vi "写入数据.vi"(6 "数据属性":variant, 8 "错误输入（无错误）":errorcluster, 11 "测试数据":dbl[][](array[numeric])) -> (0 "错误输出":errorcluster)   [LabVIEW 2020]
uses:
  <vilib>/drjdpowell/SQLite Library/SQL Statement/SQL Statement.lvclass/SQL Statement.ctl
  <vilib>/drjdpowell/SQLite Library/SQL Connection/Open (path).vi
  <vilib>/drjdpowell/SQLite Library/SQL Statement/First Step.vi
  <vilib>/drjdpowell/SQLite Library/SQL Statement/Bind Timestamp (Real).vi
  <vilib>/drjdpowell/SQLite Library/SQL Statement/Bind Text.vi
  <vilib>/drjdpowell/SQLite Library/SQL Statement/Bind Blob.vi
  <vilib>/drjdpowell/SQLite Library/SQL Statement/Bind Integer.vi
  <vilib>/drjdpowell/SQLite Library/SQL Statement/Finalize (Property).vi
  <vilib>/drjdpowell/SQLite Library/SQL Connection/Open (string).vi
  <vilib>/drjdpowell/SQLite Library/SQL Statement/Step.vi
  <vilib>/drjdpowell/SQLite Library/SQL Statement/Bind Real.vi
  <vilib>/drjdpowell/SQLite Library/SQL Statement/Finalize.vi
  <vilib>/AdvancedString/Path To Command Line String.vi
  <vilib>/drjdpowell/SQLite Library/SQL Statement/Error Message.vi
  <vilib>/drjdpowell/SQLite Library/SQL Connection/Connection.lvclass
  <vilib>/drjdpowell/SQLite Library/SQL Statement/SQL Statement.lvclass
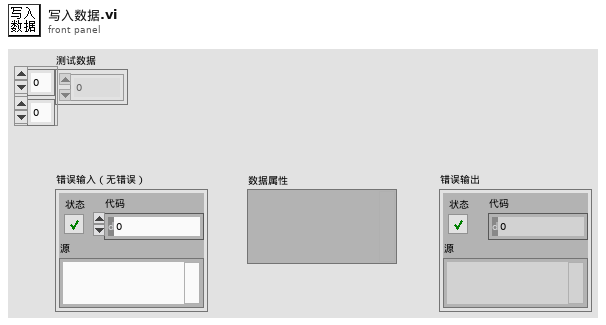
[diagram p1: front panel]
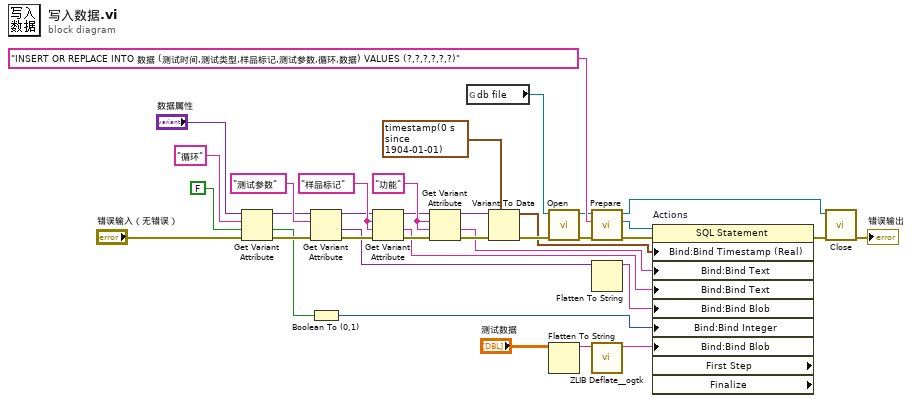
[diagram p0: block diagram]
diagram:
  w26 = "功能" ("元素")
  w33 = "样品标记" ("名称")
  n1 = Get Variant Attribute(Variant="数据属性", name="循环" ("名称"), default value (empty Variant)=FALSE, error in="错误输入（无错误）") -> (duplicate Variant=w24:variant, value=w6:bool, error out=w23:errorcluster)  [unwired: 1 out]
  n2 = Get Variant Attribute(Variant=w24, name="测试参数" ("元素"), error in=w23) -> (duplicate Variant=w22:variant, value=w8:variant, error out=w21:errorcluster)  [unwired: 1 in, 1 out]
  n3 = Boolean To (0,1)(Boolean=w6) -> (0, 1=w5:i16)
  n4 = Get Variant Attribute(Variant=w22, name=w33, default value (empty Variant)=w33, error in=w21) -> (duplicate Variant=w20:variant, value=w9:string, error out=w19:errorcluster)  [unwired: 1 out]
  n5 = Get Variant Attribute(Variant=w20, name=w26, default value (empty Variant)=w26, error in=w19) -> (duplicate Variant=w17:variant, value=w10:string, error out=w16:errorcluster)  [unwired: 1 out]
  n6 = global read "数据库.vi" "db file"() -> (w36:path)
  n7 = Variant To Data(error in=w16, type=timestamp(0 s since 1904-01-01), Variant=w17) -> (data=w11:timestamp, error out=w13:errorcluster)
  n8 = call-poly <vilib>:"Open.vi"("error in (no error)"=w13, "db file"=w36) -> ("error out"=w14:errorcluster, "SQLite Connection"=w31:refnum<class "Connection.lvclass">)  [unwired: 8 in]
  n9 = Flatten To String(anything="测试数据") -> (data string=w3:string)  [unwired: 3 in, 2 out]
  n10 = call <vilib>:"Prepare.vi"("error in (no error)"=w14, "SQL"="INSERT OR REPLACE INTO 数据 (测试时间,测试类型,样品标记,测试参数,循环,数据) VALUES (?,?,?,?,?,?)", "SQLite Connection in"=w31) -> ("error out"=w35:errorcluster, "SQL Statement"=w34:refnum<class "SQL Statement.lvclass">, "SQLite Connection"=w30:refnum<class "Connection.lvclass">)  [unwired: 4 in, 2 out]
  n11 = Flatten To String(anything=w8) -> (data string=w7:string)  [unwired: 3 in, 2 out]
  n12 = call <userlib>:"ZLIB Deflate__ogtk.vi"("input"=w3) -> ("deflated output"=w2:string)  [unwired: 4 in, 2 out]
  n13 = property on="Actions" class="SQL Statement" props=["Bind:Bind Timestamp (Real)", "Bind:Bind Text", "Bind:Bind Text", "Bind:Bind Blob", "Bind:Bind Integer", "Bind:Bind Blob", "First Step", "Finalize"](reference=w34, error in=w35, "Bind:Bind Timestamp (Real)"=w11, "Bind:Bind Text"=w10, "Bind:Bind Text"=w9, "Bind:Bind Blob"=w7, "Bind:Bind Integer"=w5, "Bind:Bind Blob"=w2) -> (error out=w29:errorcluster)  [unwired: 3 out]
  n14 = call-dynamic "Close.vi"("error in (no error)"=w29, "SQLite Connection in"=w30) -> ("error out"=→"错误输出":errorcluster)  [unwired: 9 in]
